vi "Boiler room teest.vi"() -> ()   [LabVIEW 2023]
uses:
  Heater.vi
panel:
  out "Numeric":dbl
  in  "Heater":dbl(knob) min=0.0 max=2.0 step=1.0 scale=0.0..2.0
  in  "stop":bool
  out "Thermometer":dbl(slide) scale=0.0..100.0
  in  "min temp":dbl=20.0
  in  "max temp":dbl=80.0
  in  "Automatic / Manual":bool
  out "AC":bool
  out "Heater":bool
  # "OFF"
  # "AC"
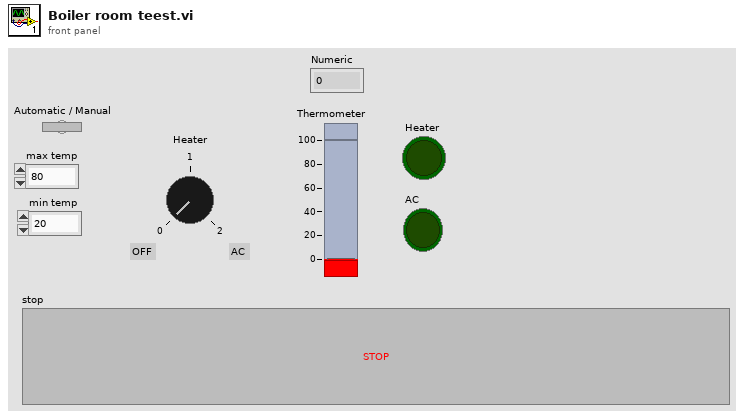
[diagram p1: front panel]
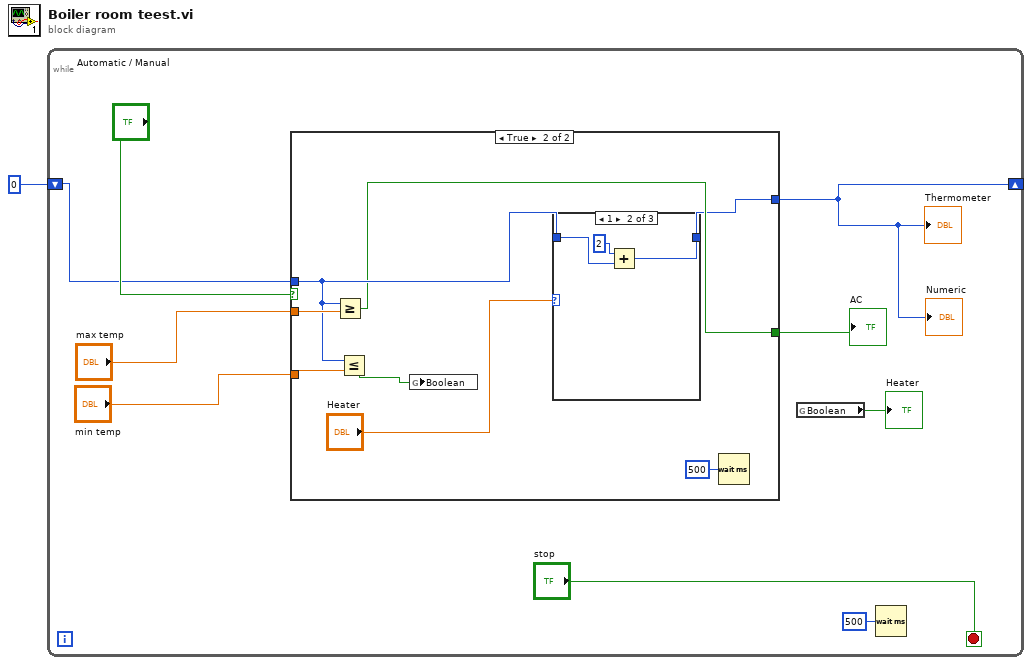
[diagram p0: block diagram]
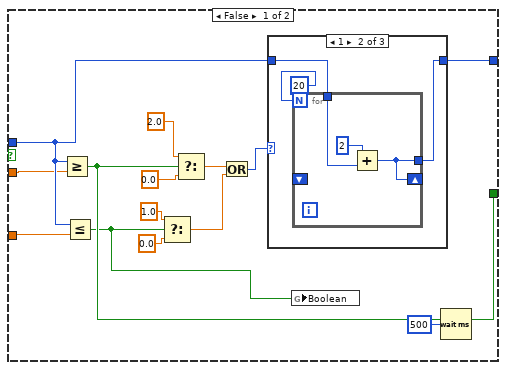
[diagram p2: hidden frame]
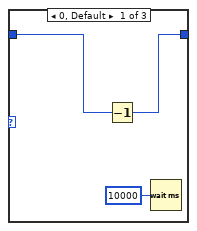
[diagram p3: hidden frame]
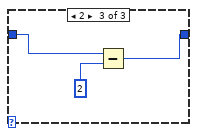
[diagram p4: hidden frame]
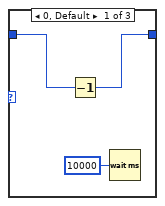
[diagram p5: hidden frame]
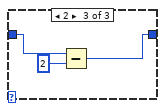
[diagram p6: hidden frame]
diagram:
  n1 = while {
    shift-right: [w4] -> _
    shift-left: 0 -> [w7]
    stop <- "stop" stop-if-true
    n2 = case shown="True" "Automatic / Manual" {
      tunnel: [w13 w40] -> w3
      tunnel: w7 -> [w16 w41]
      tunnel: "max temp" -> [w15 w43]
      tunnel: "min temp" -> [w14 w42]
      tunnel: [w18 w38] -> w4
      frame False {
        n3 = Greater Or Equal?(x=w16, y=w15) -> (x >= y?=w13:bool)
        n4 = Less Or Equal?(x=w16, y=w14) -> (x <= y?=w11:bool)
        n5 = Select(t=1.0, s=w11, f=0.0) -> (s? t:f=w12:dbl)
        n6 = Select(t=2.0, s=w13, f=0.0) -> (s? t:f=w20:dbl)
        n7 = Or(x=w20, y=w12) -> (x .or. y?=w19:i32)
        n8 = case shown="1" w19 {
          tunnel: w16 -> [w27 w29 w36]
          tunnel: [w26 w28 w35] -> w18
          frame 0, Default {
            n9 = Decrement(x=w27) -> (x-1=w26:i32)
            n10 = Wait (ms)(milliseconds to wait=u32 10000) -> ()  [unwired: 1 out]
          }
          frame 1 {
            n11 = for {
              N: 20 -> [_]
              tunnel: w29 -> [w33]
              tunnel: [w31] -> w28
              shift-right: [w31] -> _
              shift-left: _ -> [_]
              n12 = Add(x=2, y=w33) -> (x+y=w31:i32)
            }
          }
          frame 2 {
            n13 = Subtract(x=w36, y=2) -> (x-y=w35:i32)
          }
        }
        n14 = global write "Heater.vi" "Boolean"(w11) -> ()
        n15 = Wait (ms)(milliseconds to wait=u32 500) -> ()  [unwired: 1 out]
      }
      frame True {
        n16 = Greater Or Equal?(x=w41, y=w43) -> (x >= y?=w40:bool)
        n17 = Less Or Equal?(x=w41, y=w42) -> (x <= y?=w37:bool)
        n18 = global write "Heater.vi" "Boolean"(w37) -> ()
        n19 = case shown="1" "Heater" {
          tunnel: w41 -> [w47 w50 w53]
          tunnel: [w46 w49 w52] -> w38
          frame 0, Default {
            n20 = Decrement(x=w47) -> (x-1=w46:i32)
            n21 = Wait (ms)(milliseconds to wait=u32 10000) -> ()  [unwired: 1 out]
          }
          frame 1 {
            n22 = Add(x=2, y=w50) -> (x+y=w49:i32)
          }
          frame 2 {
            n23 = Subtract(x=w53, y=2) -> (x-y=w52:i32)
          }
        }
        n24 = Wait (ms)(milliseconds to wait=u32 500) -> ()  [unwired: 1 out]
      }
    }
    "AC" <- w3
    "Thermometer" <- w4
    "Numeric" <- w4
    n25 = global read "Heater.vi" "Boolean"() -> (→"Heater":bool)
    n26 = Wait (ms)(milliseconds to wait=u32 500) -> ()  [unwired: 1 out]
  }
